vi "SearchForAllTests (Folder).vi"(8 "error in (no error)":errorcluster, 10 "Inspect Recursively":bool=TRUE, 11 "Folder":path) -> (0 "error out":errorcluster, 2 "All VIs defining a test suite":path[](array[path]), 3 "All VIs defining a test (excluding those defining a suite)":path[](array[path]))   [LabVIEW 2020, in "Caraya.lvlib"]
uses:
  Caraya.lvlib
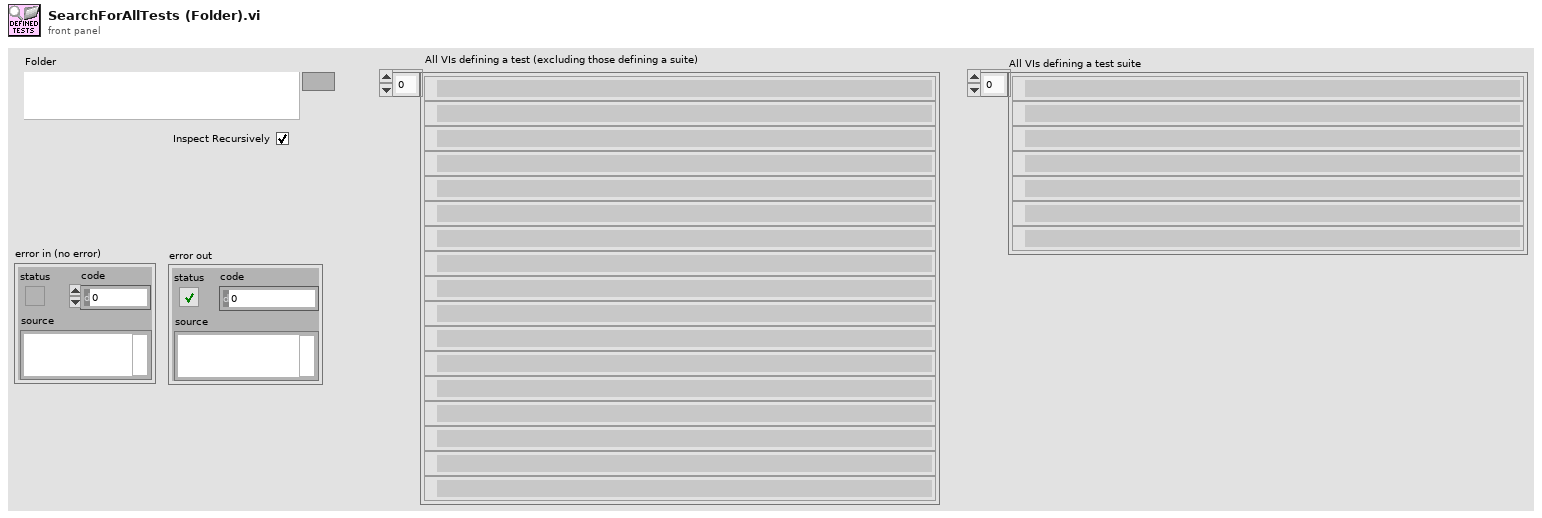
[diagram p1: front panel]
types:
  T1 = typedef "NI_FileType.lvlib/LVFileType.ctl" = enum32{"Invalid file", "Unknown type", "Instrument", "Control", "Polymorphic VI", "Project", "Library", "LVClass", "XControl", "XNode", "Shared library", ".NET assembly", "ActiveX interface", "CIN", "Run-time menu", "Palette menu", "Help file", "LLB", "XNode Edit Dependency", "Class Private Data Control", "Statechart", "MathScript .m file", "Ladder Diagram", "LVLibp", "XNode Build Dependency"}
  T2 = cluster{"path":path, "delimited name":string, "type":T1, "iState":u32, "iStyle":u16, "wStyle":u16, "buttons":u16, "viflags":u32, "viflags2":u32, "links":u32[]}[]
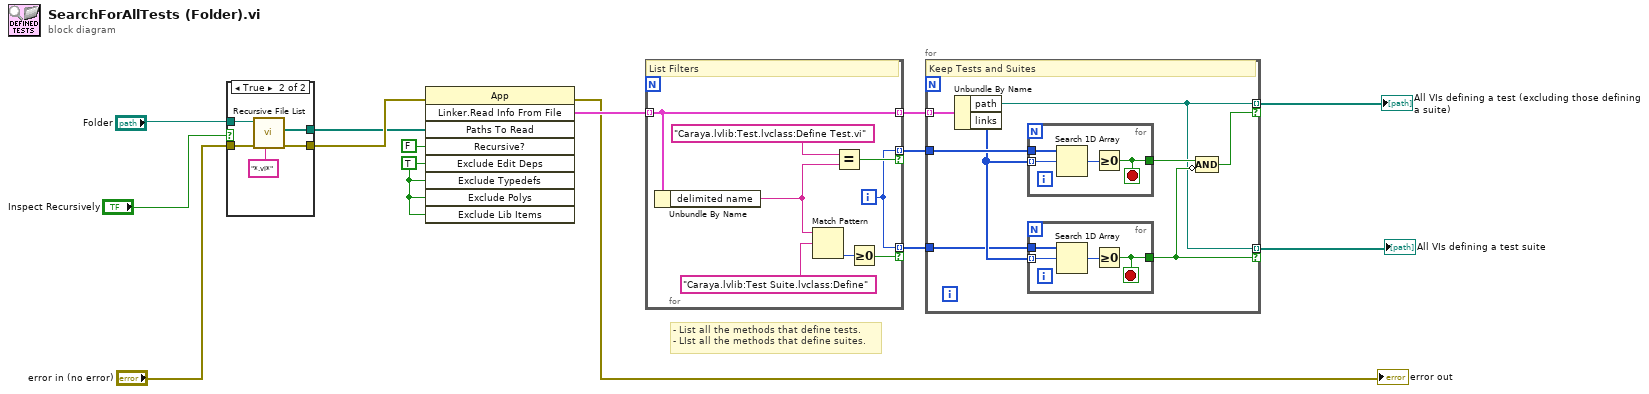
[diagram p0: block diagram]
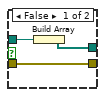
[diagram p2: hidden frame]
diagram:
  w14 = TRUE ("Exclude Edit Time Dependencies")
  # "- List all the methods that define tests.\n- LIst all the methods that define suites."
  n1 = case shown="True" "Inspect Recursively" {
    tunnel: [w15 w21] -> w10
    tunnel: "error in (no error)" -> [w15 w20]
    tunnel: "Folder" -> [w17 w19]
    tunnel: [w16 w18] -> w3
    frame False {
      n2 = Build Array(w17) -> (w16:path[])
    }
    frame True {
      n3 = call <vilib>:"Recursive File List.vi"("pattern"="*.vi*", "error in (no error)"=w20, "Folder Path"=w19) -> ("error out"=w21:errorcluster, "All Files in Dir"=w18:path[])  [unwired: 4 in, 3 out]
    }
  }
  n4 = invoke on="Invoke Node" class="App" method="Linker.Read Info From File"(error in=w10, "Paths To Read"=w3, "Recursive?"=FALSE, "Exclude Edit Deps"=w14, "Exclude Typedefs"=w14, "Exclude Polys"=w14, "Exclude Lib Items"=w14) -> (error out=→"error out":errorcluster, "Linker.Read Info From File"=w13:T2)  [unwired: 2 in, 7 out]
  n5 = for {
    tunnel: w13 -> [w25] mode=indexing
    tunnel: [w27] -> w9 mode=indexing if=w28
    tunnel: [w27] -> w8 mode=indexing if=w26
    tunnel: [w25] -> w7 mode=indexing
    i -> [w27]
    # "List Filters"
    n6 = Unbundle By Name(w25) -> ("delimited name"=w30:string)
    n7 = Match Pattern(string=w30, regular expression="Caraya.lvlib:Test Suite.lvclass:Define" ("pattern")) -> (offset past match=w29:i32)  [unwired: 1 in, 3 out]
    n8 = Equal?(x="Caraya.lvlib:Test.lvclass:Define Test.vi" ("pattern"), y=w30) -> (x = y?=w28:bool)
    n9 = Greater Or Equal To 0?(x=w29) -> (x >= 0?=w26:bool)
  }
  n10 = for {
    tunnel: w7 -> [w32] mode=indexing
    tunnel: w9 -> [w38]
    tunnel: [w31] -> w11 mode=indexing if=w33
    tunnel: w8 -> [w36]
    tunnel: [w31] -> w12 mode=indexing if=w35
    # "Keep Tests and Suites"
    n11 = Unbundle By Name(w32) -> ("path"=w31:path, "links"=w37:u32[])
    n12 = for {
      tunnel: w38 -> [w46]
      tunnel: w37 -> [w45] mode=indexing
      tunnel: [w43] -> w34
      stop <- w43 stop-if-true
      n13 = Search 1D Array(1D array=w46, element=w45) -> (index of element=w44:i32)  [unwired: 1 in]
      n14 = Greater Or Equal To 0?(x=w44) -> (x >= 0?=w43:bool)
    }
    n15 = for {
      tunnel: w36 -> [w42]
      tunnel: w37 -> [w41] mode=indexing
      tunnel: [w39] -> w35
      stop <- w39 stop-if-true
      n16 = Search 1D Array(1D array=w42, element=w41) -> (index of element=w40:i32)  [unwired: 1 in]
      n17 = Greater Or Equal To 0?(x=w40) -> (x >= 0?=w39:bool)
    }
    n18 = Compound Arithmetic op=AND(w34, invert w35) -> (w33:bool)
  }
  "All VIs defining a test (excluding those defining a suite)" <- w11
  "All VIs defining a test suite" <- w12
